vi "Assignment 5.vi"() -> ()   [LabVIEW 2021]
panel:
  in  "stop":bool
  out "Green.":bool
  out "Amber.":bool
  out "Red.":bool
  out "Green":bool
  out "Amber":bool
  out "Red":bool
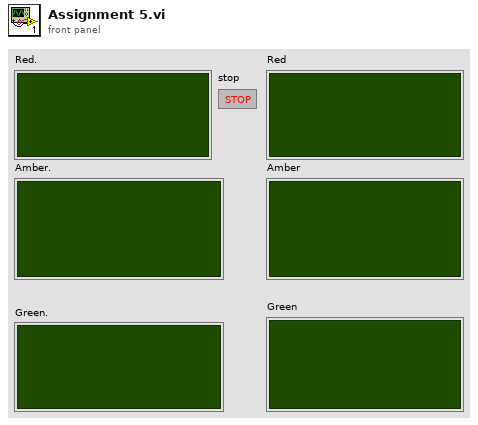
[diagram p1: front panel]
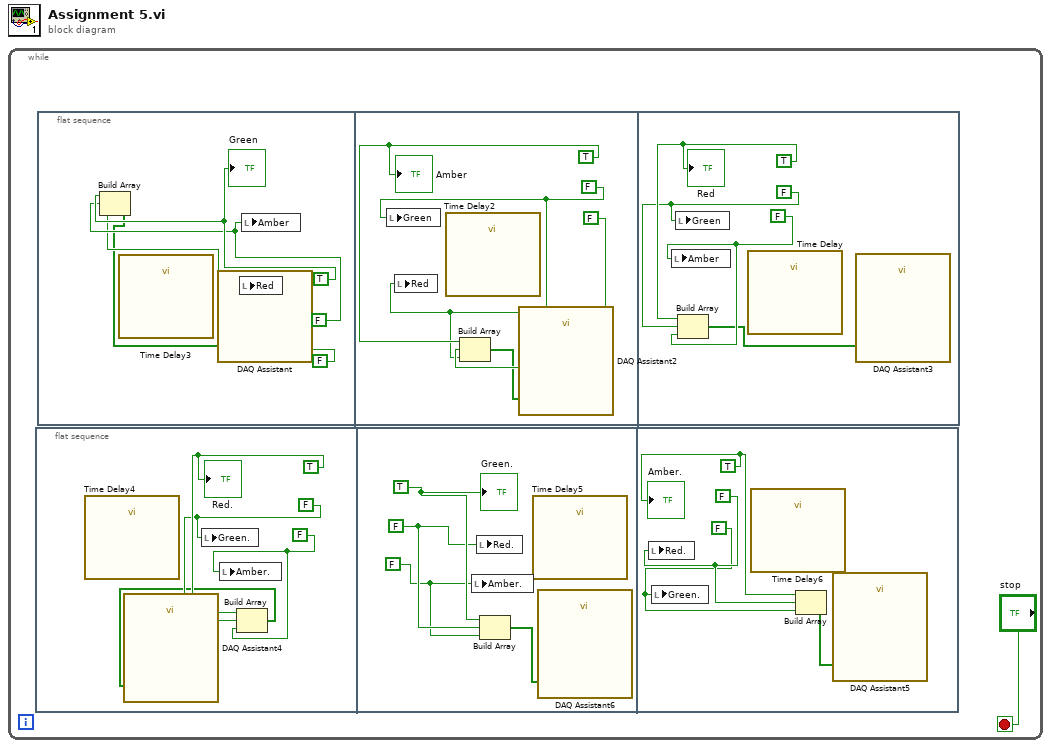
[diagram p0: block diagram]
diagram:
  n1 = while {
    stop <- "stop" stop-if-true
    n2 = flat-sequence {
      frame #0 {
        w3 = FALSE
        w4 = FALSE
        w5 = TRUE
        n3 = call "Time Delay4"() -> ()  [unwired: 11 in, 1 out]
        n4 = local write "Green."(w4) -> ()
        n5 = local write "Amber."(w3) -> ()
        n6 = Build Array(w5, w4, w3) -> (w2:bool[])
        n7 = call "DAQ Assistant4"("data"=w2) -> ()  [unwired: 17 in, 2 out]
        "Red." <- w5
      }
      frame #1 {
        w7 = FALSE
        w8 = FALSE
        w9 = TRUE
        n8 = local write "Amber."(w7) -> ()
        n9 = local write "Red."(w8) -> ()
        n10 = Build Array(w9, w8, w7) -> (w6:bool[])
        n11 = call "Time Delay5"() -> ()  [unwired: 11 in, 1 out]
        n12 = call "DAQ Assistant6"("data"=w6) -> ()  [unwired: 17 in, 2 out]
        "Green." <- w9
      }
      frame #2 {
        w11 = FALSE
        w12 = FALSE
        w13 = TRUE
        n13 = local write "Red."(w12) -> ()
        n14 = local write "Green."(w11) -> ()
        n15 = call "Time Delay6"() -> ()  [unwired: 11 in, 1 out]
        n16 = Build Array(w13, w12, w11) -> (w10:bool[])
        n17 = call "DAQ Assistant5"("data"=w10) -> ()  [unwired: 17 in, 2 out]
        "Amber." <- w13
      }
    }
    n18 = flat-sequence {
      frame #0 {
        w15 = FALSE
        w16 = FALSE
        w17 = TRUE
        n19 = Build Array(w17, w16, w15) -> (w14:bool[])
        n20 = call "Time Delay3"() -> ()  [unwired: 11 in, 1 out]
        n21 = call "DAQ Assistant"("data"=w14) -> ()  [unwired: 17 in, 2 out]
        n22 = local write "Red"(w15) -> ()
        n23 = local write "Amber"(w16) -> ()
        "Green" <- w17
      }
      frame #1 {
        w19 = FALSE
        w20 = FALSE
        w21 = TRUE
        n24 = local write "Green"(w20) -> ()
        n25 = local write "Red"(w19) -> ()
        n26 = call "Time Delay2"() -> ()  [unwired: 11 in, 1 out]
        n27 = Build Array(w21, w20, w19) -> (w18:bool[])
        n28 = call "DAQ Assistant2"("data"=w18) -> ()  [unwired: 17 in, 2 out]
        "Amber" <- w21
      }
      frame #2 {
        w23 = FALSE
        w24 = FALSE
        w25 = TRUE
        n29 = local write "Amber"(w23) -> ()
        n30 = local write "Green"(w24) -> ()
        n31 = Build Array(w25, w24, w23) -> (w22:bool[])
        n32 = call "Time Delay"() -> ()  [unwired: 11 in, 1 out]
        n33 = call "DAQ Assistant3"("data"=w22) -> ()  [unwired: 17 in, 2 out]
        "Red" <- w25
      }
    }
  }
